vi "Open MDIF File.vi"(8 "error in (no error)":errorcluster, 11 "MDIF File Path":path) -> (0 "error out":errorcluster, 3 "MDIF reference out":refnum<k24>)   [LabVIEW 2023, in "NI_HFNetworkAnalysis.lvlib"]
doc: "Open a reference to the specified MDIF file and load all its MDIF blocks into memory.\n\n<b>Note</b>\nUse <b>Get MDIF Blocks.vi</b> to retrieve the MDIF blocks from the referenced file."
uses:
  NI_HFNetworkAnalysis.lvlib
  C:/srd-semi-rfcal-software/AuxTools/STSRFFixtureCharactUtility/Source/Code Modules/Fixture/Dependencies/HFNetworkAnalysis/Support Files/NACE.Utils.Data.dll
  Support Files/NACE.Utils.Data.dll
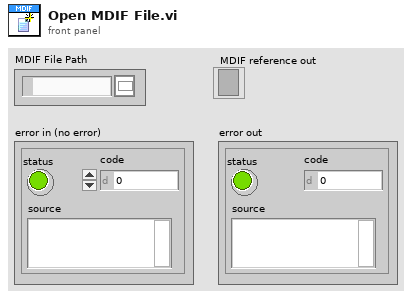
[diagram p1: front panel]
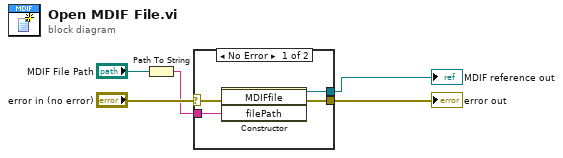
[diagram p0: block diagram]
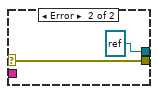
[diagram p2: hidden frame]
diagram:
  n1 = Path To String(path="MDIF File Path") -> (string=w3:string)
  n2 = case shown="No Error" "error in (no error)" {
    selector: "error in (no error)" -> [w9 w11]
    tunnel: w3 -> [w8 _]
    tunnel: [w7 w11] -> w2
    tunnel: [w6 refnum<k24> refnum ("new reference")] -> w1
    frame No Error {
      n3 = constructor class="MDIFfile"(error in=w9, "filePath"=w8) -> (reference out=w6:refnum<k24>, error out=w7:errorcluster)  [unwired: 2 in, 2 out]
    }
    frame Error {
    }
  }
  "MDIF reference out" <- w1
  "error out" <- w2
